vi "Example Callback - UVLight Callback.vi"(4 "UVLight":refnum<user-event>, 5 "Event Data":cluster{"sender":refnum<k24>, "uvLight":i64}, 6 "Control Ref":refnum<k24>, 7 "Event Common Data":T1) -> ()   [LabVIEW 2010]
uses:
  C:/tf/play/labview/Tinkerforge.dll
  Tinkerforge.dll
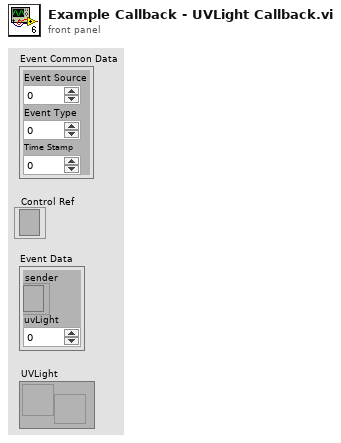
[diagram p1: front panel]
types:
  T1 = cluster{"Event Source":i32, "Event Type":u32, "Time Stamp":u32}
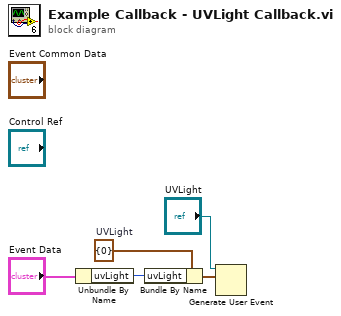
[diagram p0: block diagram]
diagram:
  w5 = cluster{"uvLight":i64} {"uvLight"=0}  # UVLight
  n1 = Unbundle By Name("Event Data") -> ("uvLight"=w4:i64)
  n2 = Bundle By Name(cluster=w5, "uvLight"=w4) -> (w1:cluster{"uvLight":i64})
  n3 = Generate User Event(user event="UVLight", event data cluster=w1) -> ()  [unwired: 1 in, 2 out]
